vi "Parse DIT & return elements.vi"(8 "error in (no error)":errorcluster, 11 "DIT string":string="<Coded Hash=5554><Public=456><n=12345>") -> (0 "error out":errorcluster, 1 "Public Key (Hex)":string, 2 "Decoded Hash value (Hex)":string="ÿÿÿÿ", 3 "n (Hex)":string="ÿÿÿÿ")   [LabVIEW 2013]
doc: "Takes the coded hash, public, and n tokens in the string and returns values.\n\nFormat of tag\n<DIT><Coded Hash=xxxxx><Public=xxxxx><n=xxxxx></DIT>"
panel:
  out "Coded hash (ASCII)":string="ÿÿÿÿ"
  # "normal display"
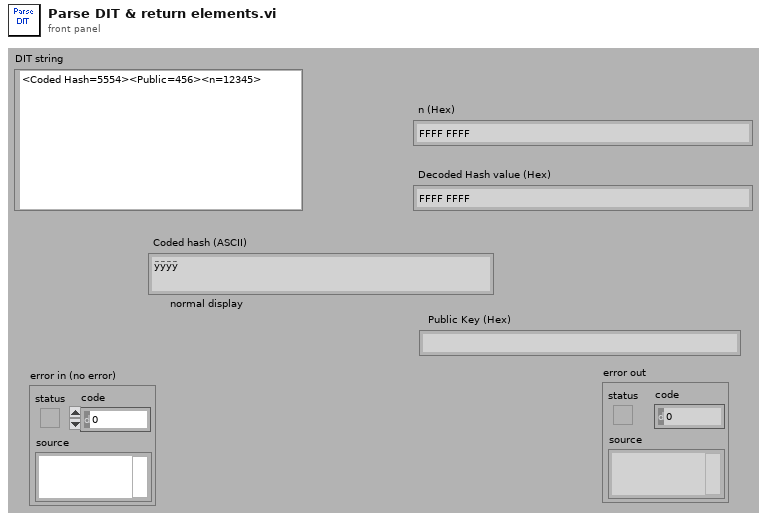
[diagram p1: front panel]
types:
  T1 = typedef "Large number - U8 array.ctl" = u8[]
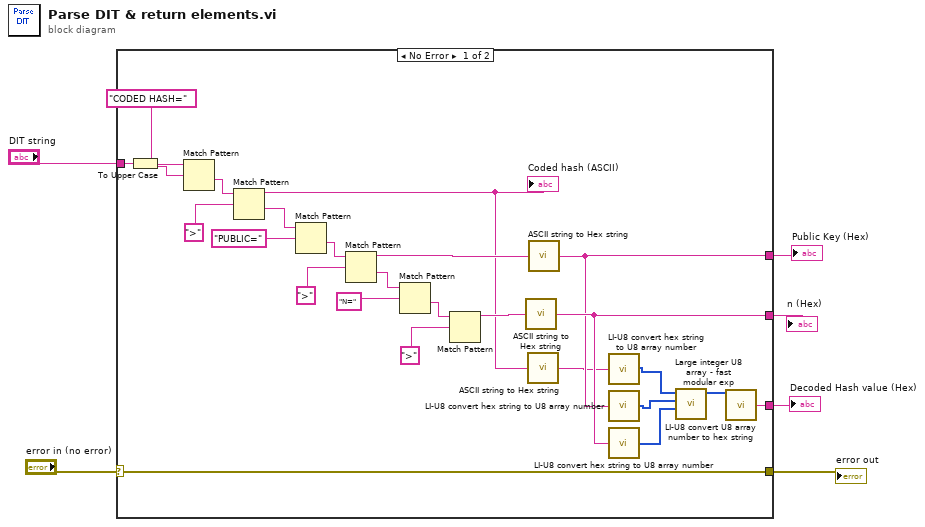
[diagram p0: block diagram]
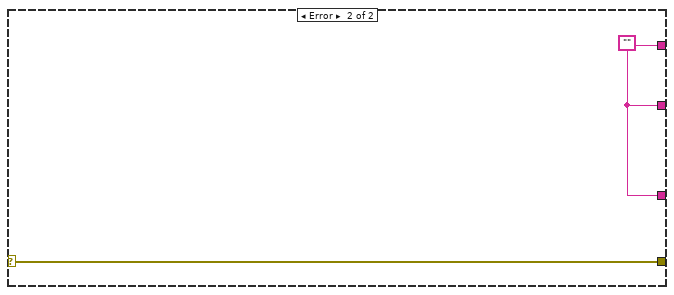
[diagram p2: hidden frame]
diagram:
  n1 = case shown="No Error" "error in (no error)" {
    selector: "error in (no error)" -> [w12 w33]
    tunnel: [w12 w33] -> w5
    tunnel: "DIT string" -> [w30 _]
    tunnel: [w9 w32] -> w3
    tunnel: [w8 w32] -> w2
    tunnel: [w13 w32] -> w1
    frame No Error {
      n2 = To Upper Case(1:w30) -> (0:w11:string)
      n3 = Match Pattern(string=w11, regular expression="CODED HASH=" ("string")) -> (after substring=w28:string)  [unwired: 4 out]
      n4 = Match Pattern(string=w28, regular expression=">") -> (before substring=w10:string, after substring=w25:string)  [unwired: 3 out]
      "Coded hash (ASCII)" <- w10
      n5 = Match Pattern(string=w25, regular expression="PUBLIC=" ("string")) -> (after substring=w27:string)  [unwired: 4 out]
      n6 = Match Pattern(string=w27, regular expression=">") -> (before substring=w19:string, after substring=w20:string)  [unwired: 3 out]
      n7 = Match Pattern(string=w20, regular expression="N=" ("string")) -> (after substring=w22:string)  [unwired: 4 out]
      n8 = Match Pattern(string=w22, regular expression=">") -> (before substring=w18:string)  [unwired: 4 out]
      n9 = call "ASCII string to Hex string.vi"("ASCII string"=w18) -> ("hex String"=w9:string)  [unwired: 4 out]
      n10 = call "ASCII string to Hex string.vi"("ASCII string"=w10) -> ("hex String"=w7:string)  [unwired: 4 out]
      n11 = call "ASCII string to Hex string.vi"("ASCII string"=w19) -> ("hex String"=w8:string)  [unwired: 4 out]
      n12 = call "LI-U8 convert hex string to U8 array number .vi"("hex string (MSD 1st)"=w7) -> ("Large number -U8"=w15:T1)  [unwired: 4 out]
      n13 = call "LI-U8 convert hex string to U8 array number .vi"("hex string (MSD 1st)"=w8) -> ("Large number -U8"=w16:T1)  [unwired: 4 out]
      n14 = call "LI-U8 convert hex string to U8 array number .vi"("hex string (MSD 1st)"=w9) -> ("Large number -U8"=w17:T1)  [unwired: 4 out]
      n15 = call "Large integer U8 array - fast modular exp.vi"("n (LI_U8)"=w17, "Exponent e (LI-U8)"=w16, "B (LI-U8)"=w15) -> ("B^e mod n"=w14:T1)  [unwired: 8 out]
      n16 = call "LI-U8 convert U8 array number to hex string.vi"("Large number -U8"=w14) -> ("hex string (MSD 1st)"=w13:string)  [unwired: 4 out]
    }
    frame Error {
      w32 = ""
    }
  }
  "n (Hex)" <- w3
  "error out" <- w5
  "Public Key (Hex)" <- w2
  "Decoded Hash value (Hex)" <- w1
